vi "H1_Density_Test_V1.vi"() -> ()   [LabVIEW 2020]
uses:
  <instrlib>/niFgen/niFgen.llb/niFgen Output Mode.ctl
  <instrlib>/niFgen/niFgen.llb/niFgen Waveform Type.ctl
  <instrlib>/niFgen/niFgen.llb/niFgen_ctl Trigger DigEdge - Edge Values (Ring).ctl
  <instrlib>/niFgen/niFgen.llb/niFgen_ctl Trigger Source Values (Ring).ctl
  <instrlib>/niFgen/niFgen.llb/niFgen Trigger Mode.ctl
  <instrlib>/niScope/Controls/niScope acquisition type.ctl
  <instrlib>/niScope/Controls/niScope trigger slope.ctl
  <instrlib>/niScope/Controls/niScope trigger source.ctl
  <vilib>/Utility/file.llb/Read Delimited Spreadsheet (DBL).vi
  <instrlib>/niFgen/niFgen.llb/niFgen Create Waveform (DBL).vi
  <instrlib>/niScope/Configure/Trigger/niScope Configure Trigger Edge.vi
  <instrlib>/niFgen/niFgen.llb/niFgen Configure Digital Edge Start Trigger.vi
  <instrlib>/niScope/Acquire/Fetch/niScope Fetch Cluster.vi
panel:
  out "Peak Amplitude 2":dbl[](array[numeric])=[0.7524058042652836, 0.7769028692719315, 0.7777042520634104, 0.7792644046349221, 0.7690737664721656, 0.7587155897528056, 0.7656206143622847, 0.7369389598529605, 0.7186154349892504, 0.700809095893297]
  out "Averaged Pulse Echo":waveform(dbl)(graph)={"t0"=timestamp(0 s since 1904-01-01), "dt"=3.3333333333333333e-06, "Y"=array[1500 elements]} caption="Waveform Graph"
  out "Frequency List (MHz)":dbl[](array[numeric])=[27.46, 27.459, 27.458, 27.457, 27.456, 27.455, 27.454, 27.453, 27.452, 27.451]
  out "Peak Amplitude 1":dbl[](array[numeric])=[0.7524058042652836, 0.7769028692719315, 0.7777042520634104, 0.7792644046349221, 0.7690737664721656, 0.7587155897528056, 0.7656206143622847, 0.7369389598529605, 0.7186154349892504, 0.700809095893297]
  in  "Pulse Train File":path=path "D:/Single 90 & 180 Degree Pulse Echo.txt"
  in  "Starting Frequency":dbl=27465000.0 caption="Frequency" format="%.4p"
  out "Scan Number":i32=2
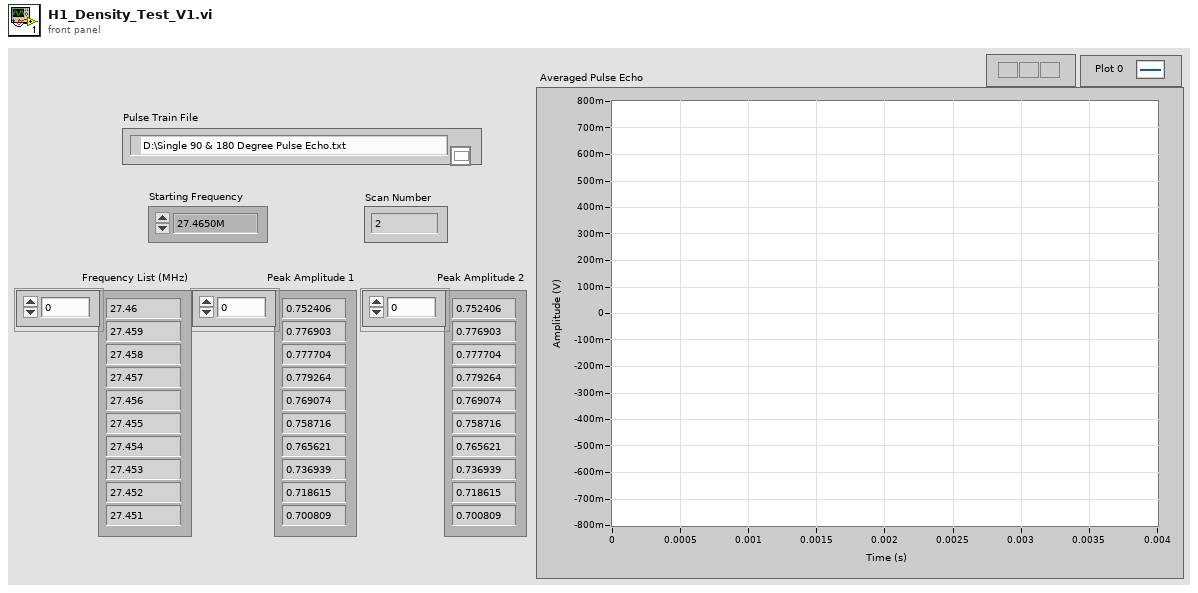
[diagram p1: front panel]
types:
  T1 = typedef "niFgen Output Mode.ctl" = u32
  T2 = typedef "niScope trigger source.ctl" = string
  T3 = typedef "niFgen_ctl Trigger Source Values (Ring).ctl" = string
  T4 = typedef "niScope trigger slope.ctl" = i32
  T5 = typedef "niScope acquisition type.ctl" = i32
  T6 = typedef "niFgen Trigger Mode.ctl" = i32
  T7 = typedef "niFgen_ctl Trigger DigEdge - Edge Values (Ring).ctl" = i32
  T8 = typedef "niFgen Waveform Type.ctl" = i32
  T9 = cluster{"relativeInitialX":dbl, "xIncrement":dbl, "wfm":dbl[]}
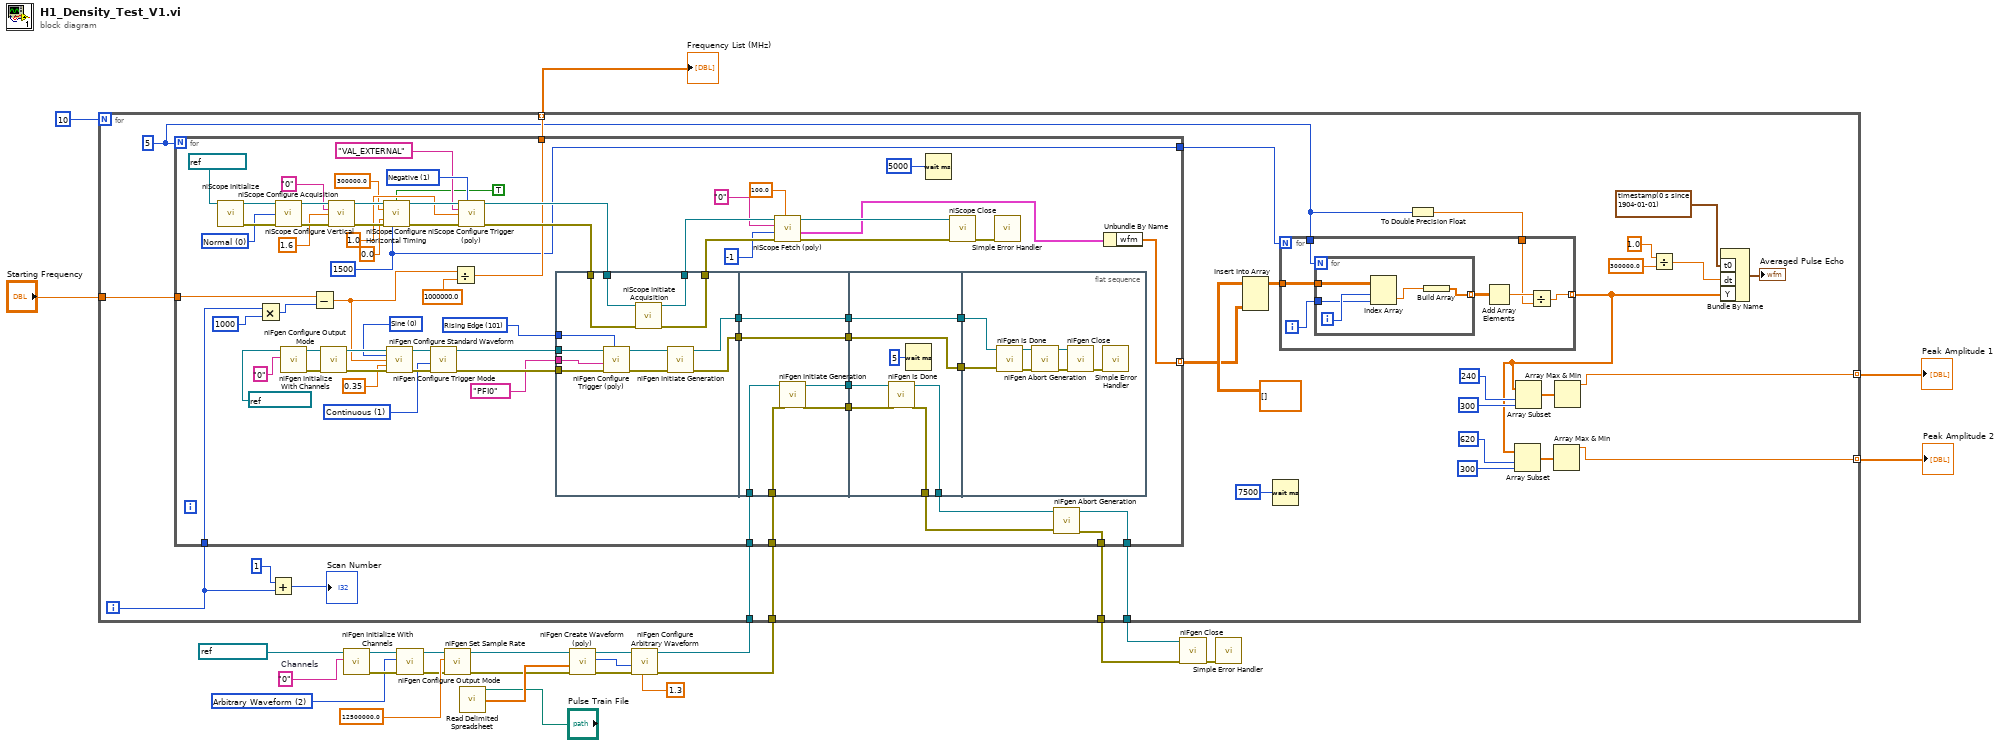
[diagram p0: block diagram]
diagram:
  w12 = "0"  # Channels
  w11 = T1 2 items=["Standard Function", "Frequency List", "Arbitrary Waveform", "Arbitrary Sequence", "Script"] ("output mode")
  n1 = call <instrlib>:"niFgen Initialize With Channels.vi"("Channel Name"=w12, "Resource Name"=refnum<k15> "PulseTrain" ("FGEN Resource Name 2")) -> ("error out"=w15:errorcluster, "Instrument Handle Out"=w16:refnum<k15>)  [unwired: 8 in]
  n2 = call <instrlib>:"niFgen Configure Output Mode.vi"("error in (no error)"=w15, "Output Mode (default: 0=Standard Function)"=w11, "Instrument Handle"=w16) -> ("error out"=w19:errorcluster, "Instrument Handle Out"=w18:refnum<k15>)  [unwired: 6 in]
  n3 = call <instrlib>:"niFgen Set Sample Rate.vi"("error in (no error)"=w19, "Sample Rate (Samp/s)"=12500000.0 ("Sample Rate"), "Instrument Handle"=w18) -> ("error out"=w22:errorcluster, "Instrument Handle Out"=w21:refnum<k15>)  [unwired: 7 in]
  n4 = call-poly <vilib>:"Read Delimited Spreadsheet.vi"("file path (dialog if empty)"="Pulse Train File") -> ("first row"=w23:dbl[])  [unwired: 9 in, 5 out]
  n5 = call-poly <instrlib>:"niFgen Create Waveform (poly).vi"("error in (no error)"=w22, "Waveform Data Array"=w23, "Instrument Handle"=w21) -> ("error out"=w25:errorcluster, "Waveform Handle"=w26:i32, "Instrument Handle Out"=w24:refnum<k15>)  [unwired: 6 in]
  n6 = call <instrlib>:"niFgen Configure Arbitrary Waveform.vi"("Gain"=1.3, "error in (no error)"=w25, "Waveform Handle"=w26, "Instrument Handle"=w24) -> ("error out"=w3:errorcluster, "Instrument Handle Out"=w4:refnum<k15>)  [unwired: 6 in]
  n7 = for {
    N: 10 -> [_]
    tunnel: [w39] -> w9 mode=indexing
    tunnel: "Starting Frequency" -> [w56]
    tunnel: [w55] -> w7 mode=indexing
    tunnel: [w54] -> w6
    tunnel: [w53] -> w5
    tunnel: w4 -> [w52]
    tunnel: w3 -> [w51]
    tunnel: [w28] -> w1 mode=indexing
    i -> [w48]
    w37 = 5 ("Number of Scans")
    n8 = for {
      N: w37 -> [_]
      tunnel: w51 -> [w119]
      tunnel: w52 -> [w118]
      tunnel: [w117] -> w54
      tunnel: [w116] -> w53
      tunnel: w56 -> [w78]
      tunnel: [w75] -> w55
      tunnel: w48 -> [w72]
      tunnel: [w71] -> w42 mode=indexing
      tunnel: [w70] -> w41
      w70 = 1500 ("min record length")
      w104 = T4 1 items=["Positive", "Negative"] ("trigger slope")
      w105 = T5 0 items=["Normal"=0, "Flex Res"=1, "DDC"=3] ("acquisition Type")
      w123 = T6 1 items=["Single", "Continuous", "Stepped", "Burst"] ("Trigger Mode (default: 1=continuous)")
      w127 = T7 101 items=["Rising Edge"=101, "Falling Edge"=102] ("Edge (Rising)")
      w128 = T8 0 items=["Sine", "Square", "Triangle", "Ramp Up", "Ramp Down", "DC", "Noise", "User"] ("Waveform")
      n9 = call <instrlib>:"niScope Initialize.vi"("resource name"=refnum<k15> "OScope") -> ("instrument handle"=w106:refnum<k15>, "error out"=w107:errorcluster)  [unwired: 13 in]
      n10 = Multiply(x=w72, y=1000) -> (x*y=w76:i32)
      n11 = call <instrlib>:"niScope Configure Acquisition.vi"("instrument handle"=w106, "acquisition Type"=w105, "error in"=w107) -> ("instrument handle out"=w109:refnum<k15>, "error out"=w110:errorcluster)  [unwired: 11 in]
      n12 = call <instrlib>:"niFgen Initialize With Channels.vi"("Channel Name"="0", "Resource Name"=refnum<k15> "FuncGen" ("Sine Wave Module")) -> ("error out"=w133:errorcluster, "Instrument Handle Out"=w136:refnum<k15>)  [unwired: 8 in]
      n13 = Subtract(x=w78, y=w76) -> (x-y=w74:dbl)
      n14 = call <instrlib>:"niFgen Configure Output Mode.vi"("error in (no error)"=w133, "Instrument Handle"=w136) -> ("error out"=w132:errorcluster, "Instrument Handle Out"=w135:refnum<k15>)  [unwired: 7 in]
      n15 = call <instrlib>:"niScope Configure Vertical.vi"("instrument handle"=w109, "channels"="0", "vertical range"=1.6, "error in"=w110) -> ("instrument handle out"=w111:refnum<k15>, "error out"=w112:errorcluster)  [unwired: 10 in]
      n16 = call <instrlib>:"niScope Configure Horizontal Timing.vi"("instrument handle"=w111, "enforce realtime"=TRUE, "min sample rate"=300000.0, "reference position"=0.0, "error in"=w112, "min record length"=w70) -> ("instrument handle out"=w113:refnum<k15>, "error out"=w114:errorcluster)  [unwired: 8 in]
      n17 = call <instrlib>:"niFgen Configure Standard Waveform.vi"("Instrument Handle"=w135, "Waveform"=w128, "Frequency"=w74, "Amplitude"=0.35, "error in (no error)"=w132) -> ("Instrument Handle Out"=w134:refnum<k15>, "error out"=w131:errorcluster)  [unwired: 9 in]
      n18 = call <instrlib>:"niFgen Configure Trigger Mode.vi"("error in (no error)"=w131, "Trigger Mode (default: 1=continuous)"=w123, "Instrument Handle"=w134) -> ("error out"=w126:errorcluster, "Instrument Handle Out"=w124:refnum<k15>)  [unwired: 7 in]
      n19 = Divide(x=w74, y=1000000.0) -> (x/y=w75:dbl)
      n20 = call-poly <instrlib>:"niScope Configure Trigger (poly).vi"("instrument handle"=w113, "trigger slope"=w104, "trigger source"=T2 "VAL_EXTERNAL", "trigger level"=1.0, "error in"=w114) -> ("instrument handle out"=w98:refnum<k15>, "error out"=w97:errorcluster)  [unwired: 9 in]
      n21 = flat-sequence {
        tunnel: w127 -> [w147]
        tunnel: w126 -> [w146]
        tunnel: T3 "PFI0" ("Source") -> [w145]
        tunnel: w124 -> [w144]
        tunnel: w98 -> [w142]
        tunnel: w97 -> [w141]
        tunnel: [w140] -> w96
        tunnel: [w139] -> w95
        tunnel: [w138] -> w85
        tunnel: [w137] -> w82
        tunnel: w119 -> [w154]
        tunnel: w118 -> [w153]
        tunnel: [w152] -> w89
        tunnel: [w151] -> w88
        tunnel: [w150] -> w86
        tunnel: w85 -> [w150]
        tunnel: [w149] -> w83
        tunnel: w82 -> [w149]
        tunnel: [w160] -> w121
        tunnel: [w159] -> w120
        tunnel: w89 -> [w158]
        tunnel: w88 -> [w157]
        tunnel: [w156] -> w87
        tunnel: w86 -> [w156]
        tunnel: [w155] -> w84
        tunnel: w83 -> [w155]
        tunnel: w87 -> [w163]
        tunnel: w84 -> [w162]
        frame #0 {
          n22 = call-poly <instrlib>:"niFgen Configure Trigger (poly).vi"("Edge (Rising)"=w147, "error in (no error)"=w146, "Source"=w145, "Instrument Handle"=w144) -> ("error out"=w143:errorcluster, "Instrument Handle Out"=w148:refnum<k15>)  [unwired: 6 in]
          n23 = call <instrlib>:"niScope Initiate Acquisition.vi"("instrument handle"=w142, "error in"=w141) -> ("instrument handle out"=w140:refnum<k15>, "error out"=w139:errorcluster)  [unwired: 12 in]
          n24 = call <instrlib>:"niFgen Initiate Generation.vi"("error in (no error)"=w143, "Instrument Handle"=w148) -> ("error out"=w137:errorcluster, "Instrument Handle Out"=w138:refnum<k15>)  [unwired: 8 in]
        }
        frame #1 {
          n25 = call <instrlib>:"niFgen Initiate Generation.vi"("error in (no error)"=w154, "Instrument Handle"=w153) -> ("error out"=w151:errorcluster, "Instrument Handle Out"=w152:refnum<k15>)  [unwired: 8 in]
        }
        frame #2 {
          n26 = call <instrlib>:"niFgen Is Done.vi"("error in (no error)"=w157, "Instrument Handle"=w158) -> ("error out"=w160:errorcluster, "Instrument Handle Out"=w159:refnum<k15>)  [unwired: 7 in, 1 out]
          n27 = Wait (ms)(milliseconds to wait=u32 5) -> ()  [unwired: 1 out]
        }
        frame #3 {
          n28 = call <instrlib>:"niFgen Is Done.vi"("error in (no error)"=w162, "Instrument Handle"=w163) -> ("error out"=w166:errorcluster, "Instrument Handle Out"=w165:refnum<k15>)  [unwired: 7 in, 1 out]
          n29 = call <instrlib>:"niFgen Abort Generation.vi"("error in (no error)"=w166, "Instrument Handle"=w165) -> ("error out"=w167:errorcluster, "Instrument Handle Out"=w168:refnum<k15>)  [unwired: 8 in]
          n30 = call <instrlib>:"niFgen Close.vi"("error in (no error)"=w167, "Instrument Handle"=w168) -> ("error out"=w164:errorcluster)  [unwired: 9 in]
          n31 = call <vilib>:"Simple Error Handler.vi"("error in (no error)"=w164) -> ()  [unwired: 4 in, 5 out]
        }
      }
      n32 = call-poly <instrlib>:"niScope Fetch (poly).vi"("timeout"=100.0, "error in"=w95, "numSamples"=-1, "channels"="0", "instrument handle"=w96) -> ("error out"=w79:errorcluster, "waveform"=w69:T9, "instrument handle out"=w80:refnum<k15>)  [unwired: 3 in, 1 out]
      n33 = Wait (ms)(milliseconds to wait=u32 5000 ("Delay Time (ms)")) -> ()  [unwired: 1 out]
      n34 = call <instrlib>:"niScope Close.vi"("instrument handle"=w80, "error in"=w79) -> ("error out"=w115:errorcluster)  [unwired: 13 in]
      n35 = call <vilib>:"Simple Error Handler.vi"("error in (no error)"=w115) -> ()  [unwired: 4 in, 5 out]
      n36 = call <instrlib>:"niFgen Abort Generation.vi"("error in (no error)"=w121, "Instrument Handle"=w120) -> ("error out"=w117:errorcluster, "Instrument Handle Out"=w116:refnum<k15>)  [unwired: 8 in]
      n37 = Unbundle By Name(w69) -> ("wfm"=w71:dbl[])
    }
    n38 = Add(x=1, y=w48) -> (x+y=→"Scan Number":i32)
    n39 = Insert Into Array(array=dbl[][] [], new element=w42) -> (w44:dbl[][])  [unwired: 2 in]
    n40 = Wait (ms)(milliseconds to wait=u32 7500 ("Delay Time (ms)")) -> ()  [unwired: 1 out]
    n41 = To Double Precision Float(number=w37) -> (double precision float=w40:dbl)
    n42 = for {
      N: w41 -> [_]
      tunnel: w44 -> [w63]
      tunnel: [w59] -> w27 mode=indexing
      tunnel: w37 -> [w58]
      tunnel: w40 -> [w57]
      i -> [w62]
      n43 = for {
        N: w58 -> [_]
        tunnel: w63 -> [w68]
        tunnel: w62 -> [w66]
        tunnel: [w64] -> w61 mode=indexing
        i -> [w67]
        n44 = Index Array(array=w68, index (row)=w67, index (col)=w66) -> (element=w65:dbl)
        n45 = Build Array(w65) -> (w64:dbl[])
      }
      n46 = Add Array Elements(numeric array=w61) -> (sum=w60:dbl)
      n47 = Divide(x=w60, y=w57) -> (x/y=w59:dbl)
    }
    n48 = Array Subset(array=w27, index=620, length=300 ("y")) -> (w31:dbl[])
    n49 = Array Subset(array=w27, index=240, length=300 ("y")) -> (w47:dbl[])
    n50 = Array Max & Min(array=w31) -> (max value=w28:dbl)  [unwired: 3 out]
    n51 = Array Max & Min(array=w47) -> (max value=w39:dbl)  [unwired: 3 out]
    n52 = Divide(x=1.0, y=300000.0) -> (x/y=w36:dbl)
    n53 = Bundle By Name("t0"=timestamp(0 s since 1904-01-01), "dt"=w36, "Y"=w27) -> (→"Averaged Pulse Echo":waveform(dbl))  [unwired: 1 in]
  }
  "Peak Amplitude 1" <- w9
  "Frequency List (MHz)" <- w7
  "Peak Amplitude 2" <- w1
  n54 = call <instrlib>:"niFgen Close.vi"("error in (no error)"=w6, "Instrument Handle"=w5) -> ("error out"=w10:errorcluster)  [unwired: 9 in]
  n55 = call <vilib>:"Simple Error Handler.vi"("error in (no error)"=w10) -> ()  [unwired: 4 in, 5 out]
